vi "save_mpi_hdf.vi"(9 "image dataset":string, 10 "Path":path, 11 "Cluster in":T1={"Magnitude meas."=[], "Phase meas."=[], "Shift meas."=[], "cw"=TRUE, "projections per image"=0, "ramp-up readouts"=0, "current sense type"="", "Number of pulses per image"=0, "Rotation enabled"=TRUE, "Rotary position"=[], "Baseline magnitude"=0.0, "Baseline phase"=0.0, "Wait readouts"=0, "Shift waveform type"="", "Shift enabled"=TRUE, "Time domain data"=[], "Motor pulse duration"=0.0, "Shift start"=0.0, "Shift stop"=0.0, "Notes"="", "Reconstructed image"=bytes[0], "Rotary encoder type"="", "Image start"=timestamp(0 s since 1904-01-01), "Image stop"=timestamp(0 s since 1904-01-01), "readouts per projection"=0, "Recon enabled"=FALSE, "Bidirectional shift"=FALSE, "Imager mode"="", "Shift delay"=0.0, "Shift frequency"=0.0, "Image time (calc)"=0.0, "Initial encoder position"=0.0, "Recon data"=[], "Trigger line values"=[], "Bed position"=0.0, "Sample image"=bytes[0], "Patch amplitude"=0.0, "Patch frequency"=0.0, "Patch phase"=0.0}) -> ()   [LabVIEW 2019]
uses:
  <vilib>/UPVI/lvhdf5/file.llb/LVH5F Operation.ctl
  <vilib>/Utility/miscctls.llb/LVRectTypeDef.ctl
  <vilib>/UPVI/lvhdf5/group.llb/H5G_obj_t.ctl
  <vilib>/UPVI/lvhdf5/dataset.llb/LVH5D Operation.ctl
  <vilib>/UPVI/lvhdf5/attribute.llb/LVH5A Operation.ctl
  <vilib>/UPVI/lvhdf5/identifier.llb/Not an HDF5 Refnum Constant.vi
  <vilib>/UPVI/lvhdf5/common.llb/To HDF5 Ref.vi
  global_variables.vi
  <vilib>/UPVI/lvhdf5/utility.llb/Select HDF5 Dialog.vi
  <vilib>/UPVI/lvhdf5/utility.llb/Select HDF5 Dialog (Object Only).vi
  <vilib>/UPVI/lvhdf5/dataset.llb/Simple H5Dwrite (Variant).vi
  <vilib>/UPVI/lvhdf5/dataset.llb/H5Dclose.vi
  <vilib>/UPVI/lvhdf5/attribute.llb/LVH5 Write Attributes.xnode
  <vilib>/UPVI/lvhdf5/library.llb/HDF5 Ref.ctl
  <vilib>/UPVI/lvhdf5/dataset.llb/Simple H5Dwrite.xnode
  <vilib>/UPVI/lvhdf5/dataset.llb/Write Dataset with Attributes.xnode
  <vilib>/Utility/VariantDataType/GetClusterInfo.vi
  <vilib>/Utility/VariantDataType/VariantType.lvlib
  <vilib>/Utility/VariantDataType/GetTypeInfo.vi
  <vilib>/UPVI/lvhdf5/attribute.llb/Cluster to Attribute Array.xnode
  <vilib>/Utility/error.llb/Error Cluster From Error Code.vi
  <vilib>/UPVI/lvhdf5/dataset.llb/OpenCreateReplace Dataset by Element Type.vi
  <vilib>/UPVI/lvhdf5/dataspace.llb/H5Sselect_hyperslab.vi
  <vilib>/UPVI/lvhdf5/dataset.llb/H5Dwrite (Variant).vi
  <vilib>/UPVI/lvhdf5/dataset.llb/H5Dget_space.vi
  <vilib>/UPVI/lvhdf5/attribute.llb/private/LVH5AwriteWDTAttrs.vi
  <vilib>/UPVI/lvhdf5/dataspace.llb/H5Sclose.vi
  <vilib>/UPVI/lvhdf5/utility.llb/Select HDF5 Dialog (File and Object).vi
  <resource>/objmgr/daqmx.rc
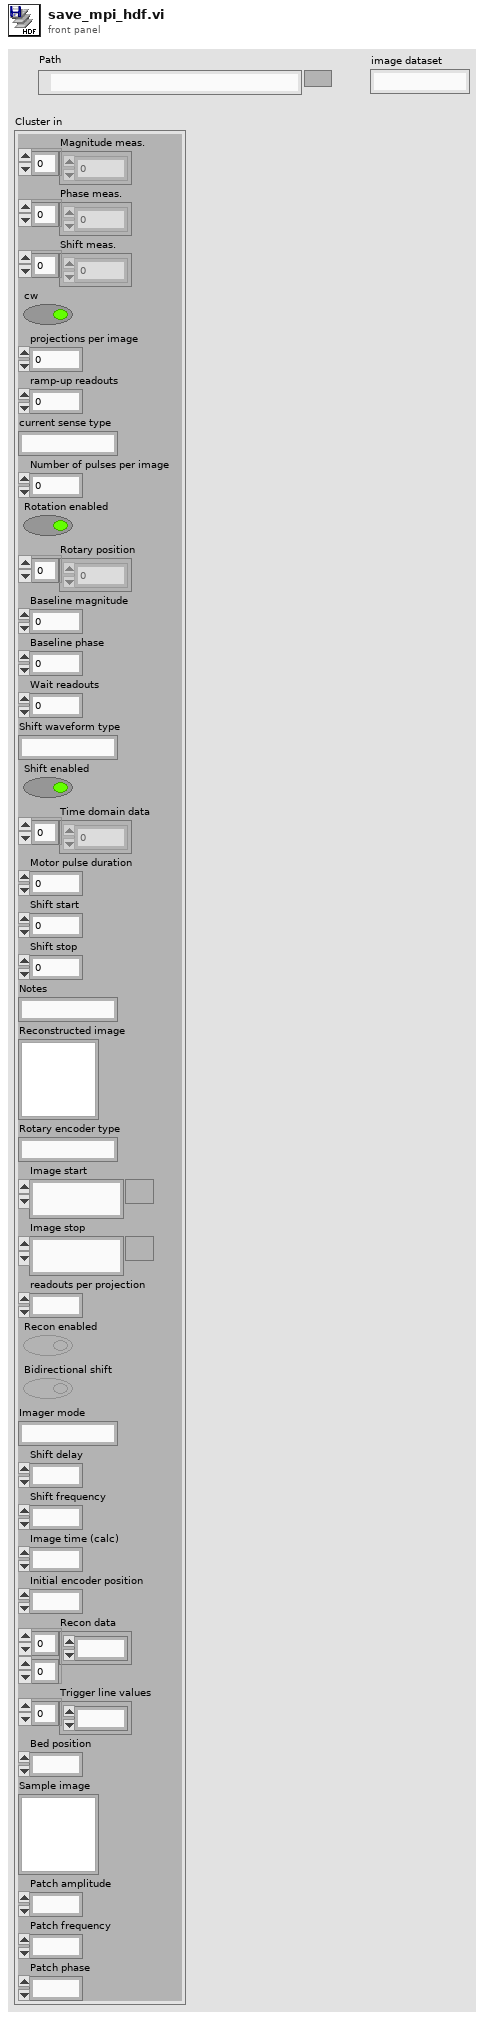
[diagram p1: front panel]
types:
  T1 = cluster{"Magnitude meas.":dbl[], "Phase meas.":dbl[], "Shift meas.":dbl[], "cw":bool, "projections per image":i32, "ramp-up readouts":i32, "current sense type":string, "Number of pulses per image":i32, "Rotation enabled":bool, "Rotary position":dbl[], "Baseline magnitude":dbl, "Baseline phase":dbl, "Wait readouts":i32, "Shift waveform type":string, "Shift enabled":bool, "Time domain data":dbl[], "Motor pulse duration":dbl, "Shift start":dbl, "Shift stop":dbl, "Notes":string, "Reconstructed image":picture, "Rotary encoder type":string, "Image start":timestamp, "Image stop":timestamp, "readouts per projection":i32, "Recon enabled":bool, "Bidirectional shift":bool, "Imager mode":string, "Shift delay":dbl, "Shift frequency":dbl, "Image time (calc)":dbl, "Initial encoder position":dbl, "Recon data":dbl[][], "Trigger line values":i32[], "Bed position":dbl, "Sample image":picture, "Patch amplitude":dbl, "Patch frequency":dbl, "Patch phase":dbl}
  T2 = typedef "LVH5F Operation.ctl" = enum16{"open", "open or create", "create or replace", "create or replace (with confirmation)", "create", "open (read only)"}
  T3 = typedef "HDF5 Ref.ctl" = refnum<k1>
  T4 = typedef "LVH5A Operation.ctl" = enum16{"open", "replace", "create", "open or create", "create or replace", "create or replace with confirmation"}
  T5 = typedef "LVRectTypeDef.ctl" = cluster{"Left":i16, "Top":i16, "Right":i16, "Bottom":i16}
  T6 = cluster{"Behavior":enum32{"Invalid", "Default", "Floating", "Floating/Auto-Hide", "Modal"}, "Position":T5, "Center":bool, "Title":string}
  T7 = typedef "LVH5D Operation.ctl" = enum16{"open", "replace", "create", "open or create", "create or replace", "create or replace with confirmation"}
  T8 = typedef "H5G_obj_t.ctl" = i32
  T9 = cluster{"Object Types (any)":T8[], "Object Pattern":string}
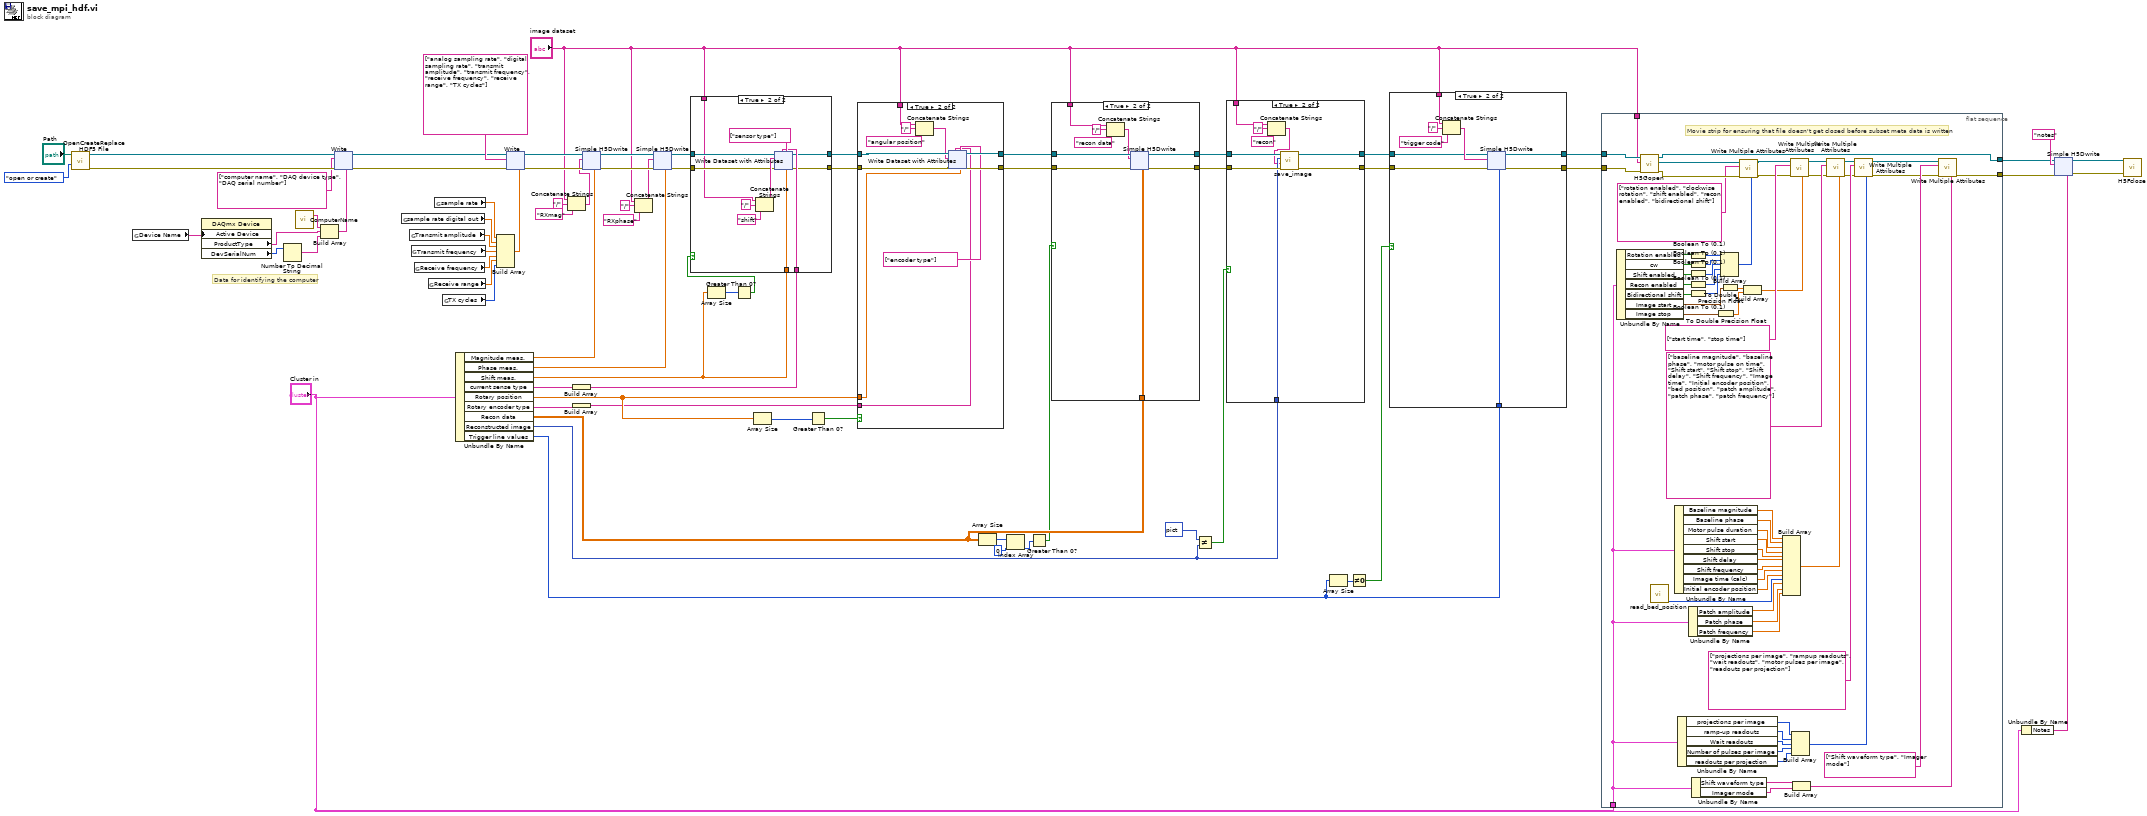
[diagram p0: block diagram]
diagram:
  # "Data for identifying the computer"
  n1 = call <vilib>:"OpenCreateReplace HDF5 File.vi"("function (open or create)"=LVH5F_Operation."open or create", "path"="Path") -> ("error out"=w67:errorcluster, "HDF5 Ref out"=w68:T3)  [unwired: 6 in]
  n2 = global read "global_variables.vi" "Device Name"() -> (w11:tag)
  n3 = property class="DAQmx Device"("Active Device"=w11) -> ("ProductType"=w71:string, "DevSerialNum"=w73:u32)  [unwired: 2 in, 2 out]
  n4 = Number To Decimal String(number=w73) -> (decimal integer string=w72:string)  [unwired: 1 in]
  n5 = call "ComputerName.vi"() -> ("String/Binary data"=w70:string)  [unwired: 4 in, 1 out]
  n6 = Build Array(w70, w71, w72) -> (w69:string[])
  n7 = xnode "Write"("HDF5 Ref"=w68, "error in (no error)"=w67, "Name(s)"=string[] ["computer name", "DAQ device type", "DAQ serial number"], "Value(s)"=w69) -> ("HDF5 Ref out"=w33:T3, "error out"=w32:errorcluster)  [unwired: 1 in]
  n8 = global read "global_variables.vi" "sample rate digital out"() -> (w65:dbl)
  n9 = global read "global_variables.vi" "Transmit amplitude"() -> (w64:dbl)
  n10 = global read "global_variables.vi" "Transmit frequency"() -> (w63:dbl)
  n11 = global read "global_variables.vi" "Receive frequency"() -> (w36:dbl)
  n12 = global read "global_variables.vi" "Receive range"() -> (w35:dbl)
  n13 = global read "global_variables.vi" "sample rate"() -> (w66:dbl)
  n14 = global read "global_variables.vi" "TX cycles"() -> (w34:i32)
  n15 = Unbundle By Name("Cluster in") -> ("Magnitude meas."=w54:dbl[], "Phase meas."=w48:dbl[], "Shift meas."=w29:dbl[], "current sense type"=w45:string, "Rotary position"=w40:dbl[], "Rotary encoder type"=w43:string, "Recon data"=w16:dbl[][], "Reconstructed image"=w19:picture, "Trigger line values"=w2:i32[])
  n16 = Build Array(w66, w65, w64, w63, w36, w35, w34) -> (w60:dbl[])
  n17 = xnode "Write"("HDF5 Ref"=w33, "error in (no error)"=w32, "Name(s)"=string[] ["analog sampling rate", "digital sampling rate", "transmit amplitude", "transmit frequency", "receive frequency", "receive range", "TX cycles"], "Value(s)"=w60) -> ("HDF5 Ref out"=w57:T3, "error out"=w56:errorcluster)  [unwired: 1 in]
  n18 = Concatenate Strings("image dataset", "/" ("string"), "RXmag" ("string")) -> (w55:string)
  n19 = Build Array(w45) -> (w44:string[])
  n20 = Build Array(w43) -> (w37:string[])
  n21 = xnode "Simple H5Dwrite"("Dataset Path"=w55, "error in (no error)"=w56, "HDF5 Path or Ref"=w57, "Data"=w54) -> ("HDF5 Ref out"=w53:T3, "error out"=w52:errorcluster)  [unwired: 4 in, 1 out]
  n22 = Concatenate Strings("image dataset", "/" ("string"), "RXphase" ("string")) -> (w49:string)
  n23 = xnode "Simple H5Dwrite"("Dataset Path"=w49, "error in (no error)"=w52, "HDF5 Path or Ref"=w53, "Data"=w48) -> ("HDF5 Ref out"=w47:T3, "error out"=w46:errorcluster)  [unwired: 4 in, 1 out]
  n24 = Array Size(array=w29) -> (size(s)=w30:i32)
  n25 = Greater Than 0?(x=w30) -> (x > 0?=w31:bool)
  n26 = case shown="True" w31 {
    tunnel: w47 -> [w77 w85]
    tunnel: w46 -> [w76 w84]
    tunnel: w29 -> [_ w83]
    tunnel: w44 -> [_ w81]
    tunnel: [w77 w80] -> w42
    tunnel: [w76 w79] -> w41
    tunnel: "image dataset" -> [_ w78]
    frame False {
    }
    frame True {
      n27 = Concatenate Strings(w78, "/" ("string"), "shift" ("string")) -> (w88:string)
      n28 = xnode "Write Dataset with Attributes"("Dataset Path"=w88, "error in (no error)"=w84, "HDF5 Path or Ref"=w85, "Attribute Name(s)"=string[] ["sensor type"], "Attribute Value(s)"=w81, "Data"=w83) -> ("HDF5 Ref out"=w80:T3, "error out"=w79:errorcluster)  [unwired: 2 in, 1 out]
    }
  }
  n29 = Array Size(array=w40) -> (size(s)=w39:i32)
  n30 = Greater Than 0?(x=w39) -> (x > 0?=w38:bool)
  n31 = case shown="True" w38 {
    tunnel: w42 -> [w384 w392]
    tunnel: w41 -> [w383 w391]
    tunnel: [w384 w390] -> w25
    tunnel: [w383 w389] -> w24
    tunnel: w40 -> [_ w386]
    tunnel: "image dataset" -> [_ w393]
    tunnel: w37 -> [_ w385]
    frame False {
    }
    frame True {
      n32 = Concatenate Strings(w393, "/" ("string"), "angular position" ("string")) -> (w387:string)
      n33 = xnode "Write Dataset with Attributes"("Dataset Path"=w387, "error in (no error)"=w391, "HDF5 Path or Ref"=w392, "Attribute Name(s)"=string[] ["encoder type"], "Attribute Value(s)"=w385, "Data"=w386) -> ("HDF5 Ref out"=w390:T3, "error out"=w389:errorcluster)  [unwired: 2 in, 1 out]
    }
  }
  n34 = Array Size(array=w16) -> (size(s)=w15:i32[])
  n35 = Index Array(array=w15, index=0) -> (element=w13:i32)
  n36 = Greater Than 0?(x=w13) -> (x > 0?=w12:bool)
  n37 = case shown="True" w12 {
    tunnel: [w691 w700] -> w23
    tunnel: [w690 w699] -> w22
    tunnel: w25 -> [w691 w698]
    tunnel: w24 -> [w690 w697]
    tunnel: "image dataset" -> [_ w693]
    tunnel: w16 -> [_ w692]
    frame False {
    }
    frame True {
      n38 = Concatenate Strings(w693, "/" ("string"), "recon data" ("string")) -> (w694:string)
      n39 = xnode "Simple H5Dwrite"("Dataset Path"=w694, "error in (no error)"=w697, "HDF5 Path or Ref"=w698, "Data"=w692) -> ("HDF5 Ref out"=w700:T3, "error out"=w699:errorcluster)  [unwired: 4 in, 1 out]
    }
  }
  n40 = Not Equal?(x=picture data[5B] ("Reconstructed image"), y=w19) -> (x != y?=w20:bool)
  n41 = case shown="True" w20 {
    tunnel: w23 -> [w904 w913]
    tunnel: [w904 w912] -> w9
    tunnel: [w903 w911] -> w8
    tunnel: w22 -> [w903 w910]
    tunnel: w19 -> [_ w909]
    tunnel: "image dataset" -> [_ w906]
    frame False {
    }
    frame True {
      n42 = Concatenate Strings(w906, "/" ("string"), "recon" ("string")) -> (w905:string)
      n43 = call "save_image.vi"("error in (no error)"=w910, "dset_name"=w905, "picture"=w909, "HDF5 Ref"=w913) -> ("error out"=w911:errorcluster, "HDF5 Ref out"=w912:T3)  [unwired: 6 in]
    }
  }
  n44 = Array Size(array=w2) -> (size(s)=w4:i32)
  n45 = Not Equal To 0?(x=w4) -> (x != 0?=w3:bool)
  n46 = case shown="True" w3 {
    tunnel: w9 -> [w915 w920]
    tunnel: w8 -> [w914 w921]
    tunnel: [w915 w919] -> w7
    tunnel: [w914 w918] -> w6
    tunnel: "image dataset" -> [_ w917]
    tunnel: w2 -> [_ w916]
    frame False {
    }
    frame True {
      n47 = Concatenate Strings(w917, "/" ("string"), "trigger code" ("string")) -> (w922:string)
      n48 = xnode "Simple H5Dwrite"("Dataset Path"=w922, "error in (no error)"=w921, "HDF5 Path or Ref"=w920, "Data"=w916) -> ("HDF5 Ref out"=w919:T3, "error out"=w918:errorcluster)  [unwired: 4 in, 1 out]
    }
  }
  n49 = flat-sequence {
    tunnel: w6 -> [w1179]
    tunnel: w7 -> [w1186]
    tunnel: "Cluster in" -> [w1130]
    tunnel: "image dataset" -> [w1185]
    tunnel: [w1161] -> w28
    tunnel: [w1163] -> w10
    frame #0 {
      # "Movie strip for ensuring that file doesn't get closed before subset meta data is written"
      n50 = Unbundle By Name(w1130) -> ("Rotation enabled"=w1141:bool, "cw"=w1138:bool, "Shift enabled"=w1137:bool, "Recon enabled"=w1135:bool, "Bidirectional shift"=w1133:bool, "Image start"=w1178:timestamp, "Image stop"=w1175:timestamp)
      n51 = call <vilib>:"H5Gopen.vi"("error in (no error)"=w1179, "Name"=w1185, "HDF5 Ref"=w1186) -> ("error out"=w1144:errorcluster, "HDF5 Group Ref"=w1147:T3, "HDF5 Ref out"=w1163:T3)  [unwired: 4 in]
      n52 = call "read_bed_position.vi"() -> ("Absolute position (pulses)"=w1131:i32)  [unwired: 11 in]
      n53 = Unbundle By Name(w1130) -> ("Baseline magnitude"=w1184:dbl, "Baseline phase"=w1183:dbl, "Motor pulse duration"=w1182:dbl, "Shift start"=w1181:dbl, "Shift stop"=w1180:dbl, "Shift delay"=w1168:dbl, "Shift frequency"=w1167:dbl, "Image time (calc)"=w1166:dbl, "Initial encoder position"=w1164:dbl)
      n54 = Unbundle By Name(w1130) -> ("projections per image"=w1174:i32, "ramp-up readouts"=w1173:i32, "Wait readouts"=w1172:i32, "Number of pulses per image"=w1171:i32, "readouts per projection"=w1169:i32)
      n55 = Unbundle By Name(w1130) -> ("Patch amplitude"=w1127:dbl, "Patch phase"=w1128:dbl, "Patch frequency"=w1129:dbl)
      n56 = Boolean To (0,1)(Boolean=w1141) -> (0, 1=w1140:i16)
      n57 = Boolean To (0,1)(Boolean=w1138) -> (0, 1=w1139:i16)
      n58 = Boolean To (0,1)(Boolean=w1137) -> (0, 1=w1136:i16)
      n59 = Boolean To (0,1)(Boolean=w1135) -> (0, 1=w1134:i16)
      n60 = Boolean To (0,1)(Boolean=w1133) -> (0, 1=w1132:i16)
      n61 = Unbundle By Name(w1130) -> ("Shift waveform type"=w1170:string, "Imager mode"=w1165:string)
      n62 = To Double Precision Float(number=w1175) -> (double precision float=w1176:dbl)
      n63 = Build Array(w1140, w1139, w1136, w1134, w1132) -> (w1142:i16[])
      n64 = To Double Precision Float(number=w1178) -> (double precision float=w1177:dbl)
      n65 = call <vilib>:"Write Multiple Attributes.vi"("Values"=w1142, "error in (no error)"=w1144, "Names"=string[] ["rotation enabled", "clockwise rotation", "shift enabled", "recon enabled", "bidirectional shift"] ("Name(s)"), "HDF5 Ref"=w1147) -> ("error out"=w1145:errorcluster, "HDF5 Ref out"=w1146:T3)  [unwired: 4 in]
      n66 = Build Array(w1177, w1176) -> (w1148:dbl[])
      n67 = Build Array(w1184, w1183, w1182, w1181, w1180, w1168, w1167, w1166, w1164, w1131, w1127, w1128, w1129) -> (w1152:dbl[])
      n68 = call <vilib>:"Write Multiple Attributes.vi"("Values"=w1148, "error in (no error)"=w1145, "Names"=string[] ["start time", "stop time"] ("Name(s)"), "HDF5 Ref"=w1146) -> ("error out"=w1150:errorcluster, "HDF5 Ref out"=w1151:T3)  [unwired: 4 in]
      n69 = Build Array(w1174, w1173, w1172, w1171, w1169) -> (w1156:i32[])
      n70 = Build Array(w1170, w1165) -> (w1160:string[])
      n71 = call <vilib>:"Write Multiple Attributes.vi"("Values"=w1152, "error in (no error)"=w1150, "Names"=string[] ["baseline magnitude", "baseline phase", "motor pulse on time", "Shift start", "Shift stop", "Shift delay", "Shift frequency", "Image time", "Initial encoder position", "bed position", "patch amplitude", "patch phase", "patch frequency"] ("Name(s)"), "HDF5 Ref"=w1151) -> ("error out"=w1154:errorcluster, "HDF5 Ref out"=w1155:T3)  [unwired: 4 in]
      n72 = call <vilib>:"Write Multiple Attributes.vi"("Values"=w1156, "error in (no error)"=w1154, "Names"=string[] ["projections per image", "rampup readouts", "wait readouts", "motor pulses per image", "readouts per projection"] ("Name(s)"), "HDF5 Ref"=w1155) -> ("error out"=w1157:errorcluster, "HDF5 Ref out"=w1159:T3)  [unwired: 4 in]
      n73 = call <vilib>:"Write Multiple Attributes.vi"("Values"=w1160, "error in (no error)"=w1157, "Names"=string[] ["Shift waveform type", "Imager mode"] ("Name(s)"), "HDF5 Ref"=w1159) -> ("error out"=w1161:errorcluster)  [unwired: 4 in, 1 out]
    }
  }
  n74 = Unbundle By Name("Cluster in") -> ("Notes"=w26:string)
  n75 = xnode "Simple H5Dwrite"("Dataset Path"="notes", "error in (no error)"=w28, "HDF5 Path or Ref"=w10, "Data"=w26) -> ("HDF5 Ref out"=w18:T3, "error out"=w17:errorcluster)  [unwired: 4 in, 1 out]
  n76 = call <vilib>:"H5Fclose.vi"("error in (no error)"=w17, "HDF5 Ref"=w18) -> ()  [unwired: 7 in, 1 out]
